vi "Read Checkweighin Threshold.vi"(8 "error in (no error)":errorcluster, 10 "Lower Limit(T)/Upper Limit (F)":bool, 11 "VISA resource name":refnum<visa-resource-name>) -> (0 "error out":errorcluster, 1 "Threshold Unit":string, 2 "Threshold Value":dbl, 3 "VISA resource name out":refnum<visa-resource-name>)   [LabVIEW 2017, in "RadWag balances and scales.lvlib"]
doc: "Reads current values of checkweighin thresholds."
uses:
  <instrlib>/Prev/RadWag Continuous Read Folder/RadWag balances and scales.lvlib
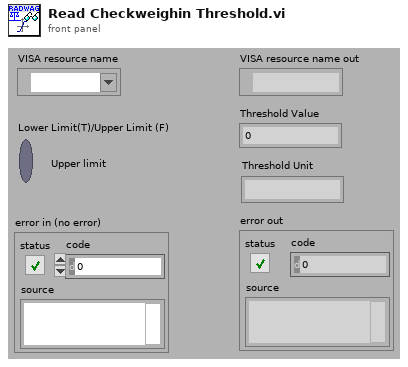
[diagram p1: front panel]
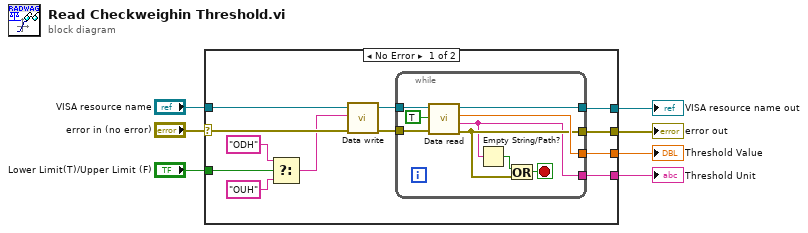
[diagram p0: block diagram]
diagram:
  n1 = case shown="No Error" "error in (no error)" {
    selector: "error in (no error)" -> [w14 w29]
    tunnel: "Lower Limit(T)/Upper Limit (F)" -> [w13 _]
    tunnel: "VISA resource name" -> [w17 w30]
    tunnel: [w16 w30] -> w4
    tunnel: [w15 w29] -> w3
    tunnel: [w9 _] -> w2
    tunnel: [w8 _] -> w1
    frame No Error {
      n2 = Select(t="ODH" ("ID"), s=w13, f="OUH" ("ID")) -> (s? t:f=w10:string)
      n3 = call <instrlib>:"Data write.vi"("error in (no error)"=w14, "ID"=w10, "VISA resource name"=w17) -> ("error out"=w18:errorcluster, "VISA resource name out"=w19:refnum<visa-resource-name>)  [unwired: 7 in]
      n4 = while {
        tunnel: w19 -> [w28]
        tunnel: w18 -> [w27]
        tunnel: [w26] -> w16
        tunnel: [w22] -> w15
        tunnel: [w23] -> w9
        tunnel: [w20] -> w8
        stop <- w25 stop-if-true
        n5 = call <instrlib>:"Data read.vi"("error in (no error)"=w27, "Decode Status (F)/ Decode Data (T)"=TRUE, "VISA resource name"=w28) -> ("error out"=w22:errorcluster, "Unit"=w20:string, "Value"=w23:dbl, "VISA resource name out"=w26:refnum<visa-resource-name>)  [unwired: 2 in, 3 out]
        n6 = Empty String/Path?(string/path=w20) -> (empty?=w21:bool)
        n7 = Or(x=w21, y=w22) -> (x .or. y?=w25:bool)
      }
    }
    frame Error {
    }
  }
  "VISA resource name out" <- w4
  "error out" <- w3
  "Threshold Value" <- w2
  "Threshold Unit" <- w1
